vi "Do.vi"(8 "error in (no error)":errorcluster, 10 "Actor in":refnum<class "Actor.lvclass">, 11 "DIO Actor Msg":refnum<class "DIO Actor Msg.lvclass">) -> (0 "error out":errorcluster, 2 "Actor out":refnum<class "Actor.lvclass">)   [LabVIEW 2024, in "DIO Actor.lvlib" / "DIO Actor Msg.lvclass"]
doc: "(<B>Filename</B>: Actor Framework.lvlib:Message.lvclass:Do.vi)\n\nDefines what a message does when it is received by an actor. Generally, a message instructs an actor to invoke one of its methods. By default, this method does nothing. A child class must override it to define behavior. Create a child class by using the Actor Framework Message Maker dialog box."
uses:
  DIO Actor Msg.lvclass
  <vilib>/ActorFramework/Actor/Actor.lvclass
  Actor/DIO.lvclass
  C:/Program Files (x86)/National Instruments/LabVIEW 2024/vi.lib/ActorFramework/Actor/Actor.lvclass
  DIO Actor Msg.lvclass/DIO Actor Msg.ctl
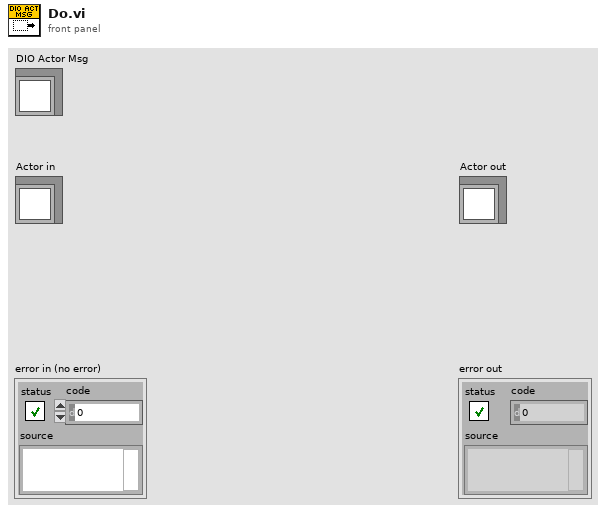
[diagram p1: front panel]
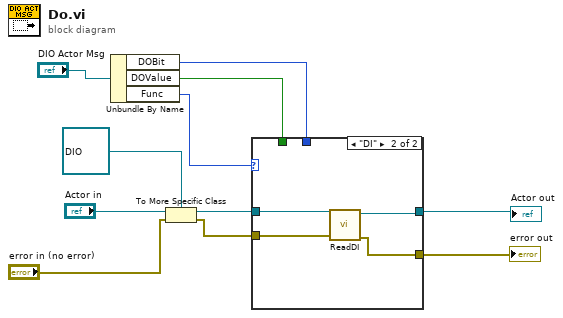
[diagram p0: block diagram]
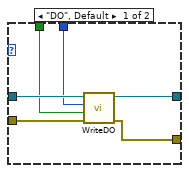
[diagram p2: hidden frame]
diagram:
  n1 = Unbundle By Name("DIO Actor Msg") -> ("DOBit"=w6:u8, "DOValue"=w5:bool, "Func"=w1:enum16{"DO", "DI"})
  n2 = To More Specific Class(target class=refnum<class "DIO.lvclass"> refnum ("DIO Actor.lvlib:DIO.lvclass"), reference="Actor in", error in="error in (no error)") -> (specific class reference=w7:refnum<class "DIO.lvclass">, error out=w4:errorcluster)
  n3 = case shown="\"DI\"" w1 {
    tunnel: w7 -> [w17 w21]
    tunnel: w6 -> [w16 _]
    tunnel: w5 -> [w15 _]
    tunnel: w4 -> [w14 w20]
    tunnel: [w13 w19] -> w3
    tunnel: [w12 w18] -> w2
    frame "DO", Default {
      n4 = call "WriteDO.vi"("error in (no error)"=w14, "DOValue"=w15, "DOBit"=w16, "DIO in"=w17) -> ("error out"=w12:errorcluster, "DIO out"=w13:refnum<class "DIO.lvclass">)  [unwired: 6 in]
    }
    frame "DI" {
      n5 = call "ReadDI.vi"("error in (no error)"=w20, "DIO in"=w21) -> ("error out"=w18:errorcluster, "DIO out"=w19:refnum<class "DIO.lvclass">)  [unwired: 8 in]
    }
  }
  "error out" <- w2
  "Actor out" <- w3
